vi "Manip4.vi"() -> ()   [LabVIEW 2021]
panel:
  out "millisecond timer value 2":u32
  out "Waveform Chart":i8(graph)
  out "Value":i8
  out "Boolean":bool
  in  "delay":u32
  in  "stop":bool
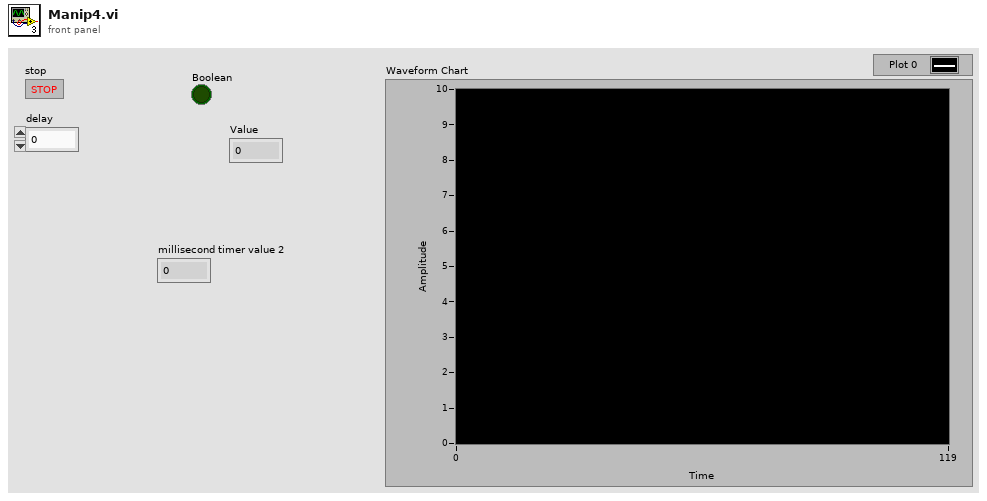
[diagram p1: front panel]
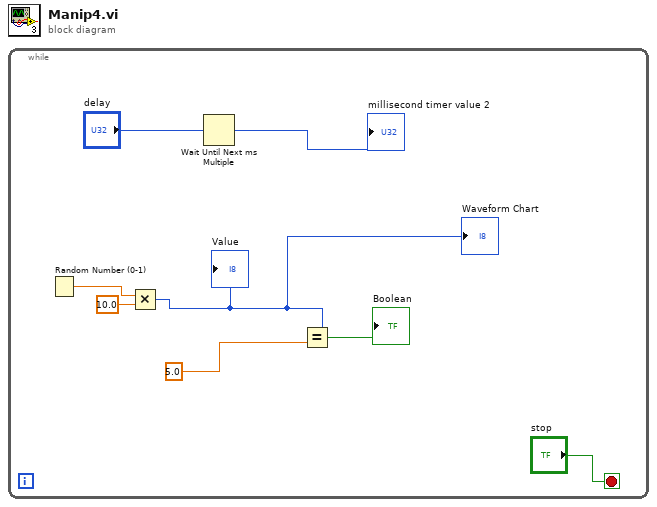
[diagram p0: block diagram]
diagram:
  n1 = while {
    stop <- "stop" stop-if-true
    n2 = Random Number (0-1)() -> (number: 0 to 1=w2:dbl)
    n3 = Multiply(x=w2, y=10.0) -> (x*y=w1:i8)
    "Value" <- w1
    "Waveform Chart" <- w1
    n4 = Wait Until Next ms Multiple(millisecond multiple="delay") -> (millisecond timer value=→"millisecond timer value 2":u32)
    n5 = Equal?(x=w1, y=5.0) -> (x = y?=→"Boolean":bool)
  }
